vi "OnTaskFailed.vi"(8 "error in (no error)":errorcluster, 9 "Device Error":errorcluster, 10 "Correlation ID":u32, 11 "AutomationContext in":refnum<class "AutomationContext.lvclass">) -> (0 "error out":errorcluster, 3 "AutomationContext out":refnum<class "AutomationContext.lvclass">)   [LabVIEW 2023, in "Automation.lvlib" / "AutomationContext.lvclass"]
uses:
  AutomationContext.lvclass
  AutomationContext.lvclass/AutomationContext.ctl
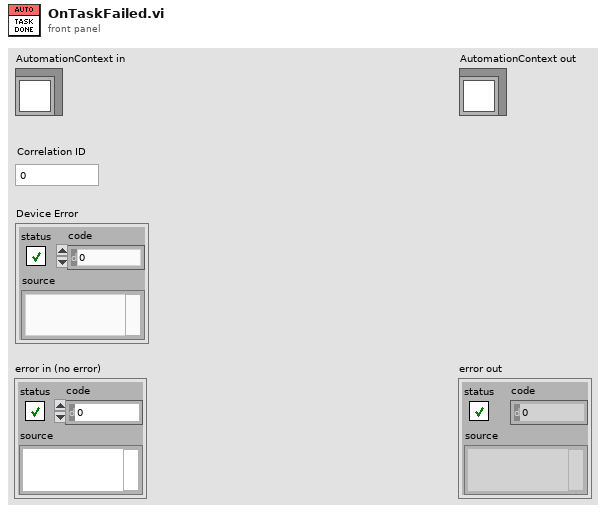
[diagram p1: front panel]
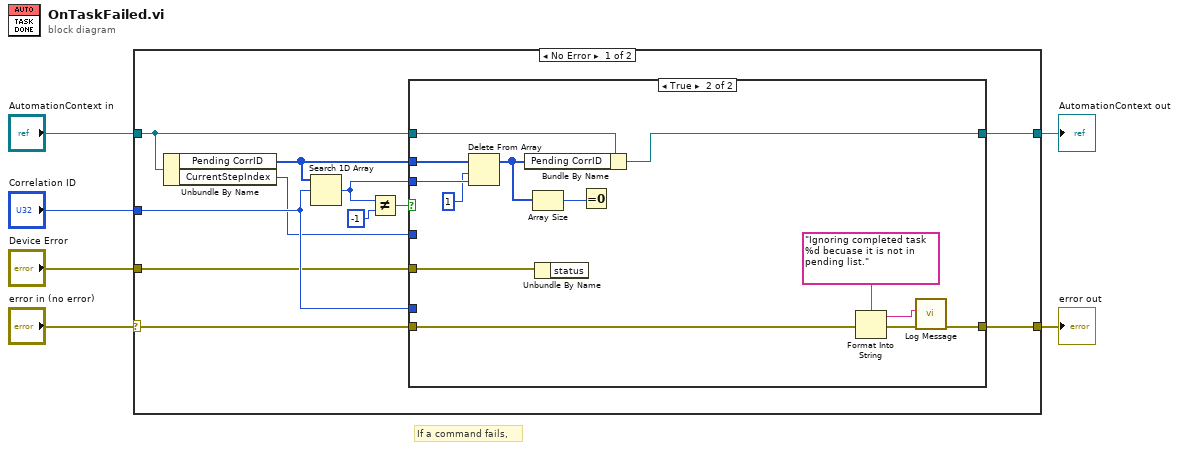
[diagram p0: block diagram]
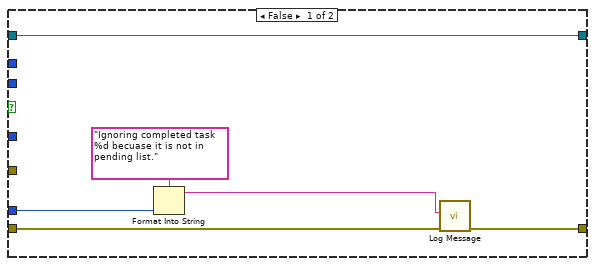
[diagram p2: hidden frame]
diagram:
  # "If a command fails,"
  n1 = case shown="No Error" "error in (no error)" {
    selector: "error in (no error)" -> [w17 w38]
    tunnel: [w16 w38] -> w5
    tunnel: [w15 w37] -> w3
    tunnel: "AutomationContext in" -> [w10 w37]
    tunnel: "Correlation ID" -> [w14 _]
    tunnel: "Device Error" -> [w7 _]
    frame No Error {
      n2 = Unbundle By Name(w10) -> ("Pending CorrID"=w9:u32[], "CurrentStepIndex"=w11:u32)
      n3 = Search 1D Array(1D array=w9, element=w14) -> (index of element=w8:i32)  [unwired: 1 in]
      n4 = Not Equal?(x=w8, y=-1) -> (x != y?=w13:bool)
      n5 = case shown="True" w13 {
        tunnel: w17 -> [w21 w25]
        tunnel: [w22 w27] -> w16
        tunnel: [w23 w30] -> w15
        tunnel: w10 -> [w23 w36]
        tunnel: w14 -> [w18 _]
        tunnel: w11 -> [_ _]
        tunnel: w9 -> [_ w35]
        tunnel: w8 -> [_ w34]
        tunnel: w7 -> [_ w24]
        frame False {
          n6 = Format Into String(format string="Ignoring completed task %d becuase it is not in pending list.", w18) -> (resulting string=w20:string)  [unwired: 2 in, 1 out]
          n7 = call "Log Message.vi"("error constant"=w21, "input"=w20) -> ("error constant 2"=w22:errorcluster)  [unwired: 8 in, 1 out]
        }
        frame True {
          n8 = Delete From Array(array=w35, length=1, index=w34) -> (array with subset deleted=w33:u32[])  [unwired: 1 out]
          n9 = Bundle By Name(cluster=w36, "Pending CorrID"=w33) -> (w30:refnum<class "AutomationContext.lvclass">)
          n10 = Array Size(array=w33) -> (size(s)=w32:i32)
          n11 = Unbundle By Name(w24) -> ()  [unwired: 1 out]
          n12 = Equal To 0?(x=w32) -> ()  [unwired: 1 out]
          n13 = Format Into String(format string="Ignoring completed task %d becuase it is not in pending list.", error in=w25) -> (resulting string=w29:string, error out=w26:errorcluster)  [unwired: 2 in]
          n14 = call "Log Message.vi"("error constant"=w26, "input"=w29) -> ("error constant 2"=w27:errorcluster)  [unwired: 8 in, 1 out]
        }
      }
    }
    frame Error {
    }
  }
  "error out" <- w5
  "AutomationContext out" <- w3
